vi "Sub01_CommandBuilder - Copy.vi"(8 "error in (no error)":errorcluster, 9 "CommandInfo":T1={"RedBall"={"Min"={"G"=0, "B"=0, "R"=160}, "Max"={"G"=160, "B"=160, "R"=255}}, "YellowBall"={"Min"={"G"=140, "B"=0, "R"=140}, "Max"={"G"=255, "B"=175, "R"=255}}, "WhiteBall"={"Min"={"G"=100, "B"=100, "R"=100}, "Max"={"G"=255, "B"=255, "R"=255}}, "BallDiameter"=11, "BackGround"={"Min"={"G"=91, "B"=202, "R"=39}, "Max"={"G"=116, "B"=255, "R"=62}}, "Border"={"Min"={"G"=0, "B"=121, "R"=0}, "Max"={"G"=42, "B"=126, "R"=14}}}, 10 "filenames":string[](array[string]), 11 "path in":path) -> (0 "error out":errorcluster, 3 "String":string)   [LabVIEW 2019]
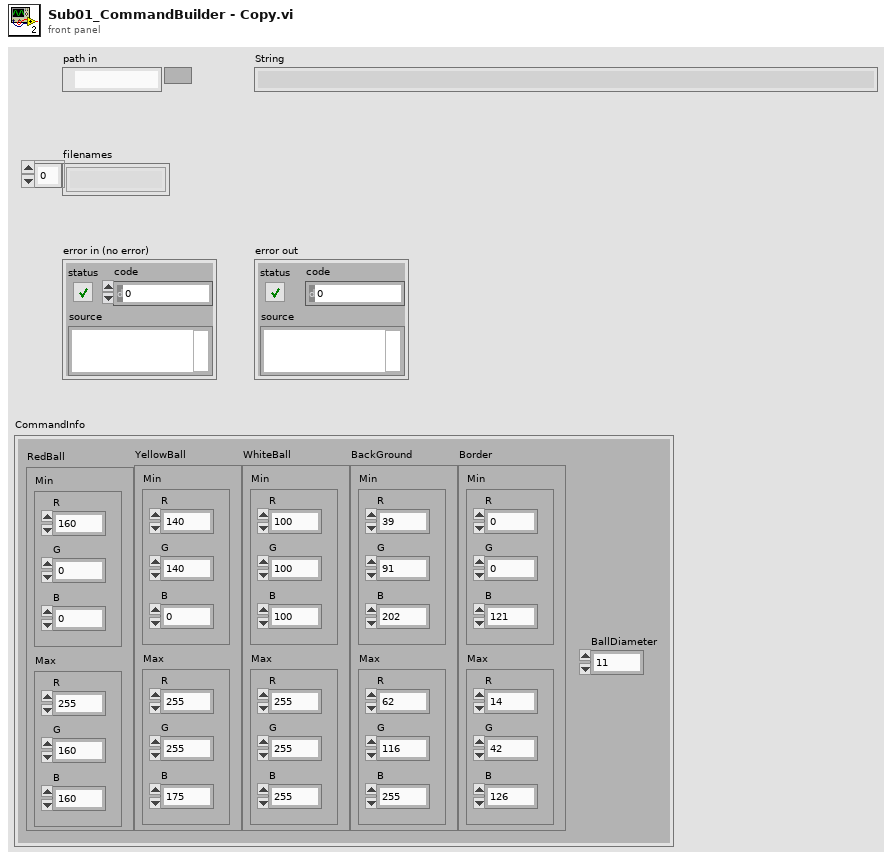
[diagram p1: front panel]
types:
  T1 = cluster{"RedBall":cluster{"Min":cluster{"G":u32, "B":u32, "R":u32}, "Max":cluster{"G":u32, "B":u32, "R":u32}}, "YellowBall":cluster{"Min":cluster{"G":u32, "B":u32, "R":u32}, "Max":cluster{"G":u32, "B":u32, "R":u32}}, "WhiteBall":cluster{"Min":cluster{"G":u32, "B":u32, "R":u32}, "Max":cluster{"G":u32, "B":u32, "R":u32}}, "BallDiameter":u32, "BackGround":cluster{"Min":cluster{"G":u32, "B":u32, "R":u32}, "Max":cluster{"G":u32, "B":u32, "R":u32}}, "Border":cluster{"Min":cluster{"G":u32, "B":u32, "R":u32}, "Max":cluster{"G":u32, "B":u32, "R":u32}}}
  T2 = cluster{"left":u32, "top":u32, "right":u32, "bottom":u32}
  T3 = typedef "imagedata.ctl" = cluster{"image type":i32, "image depth":i32, "image":u8[], "mask":u8[], "colors":u32[], "Rectangle":cluster{"left":i16, "top":i16, "right":i16, "bottom":i16}}
  T4 = cluster{"Min":cluster{"G":u32, "B":u32, "R":u32}, "Max":cluster{"G":u32, "B":u32, "R":u32}}
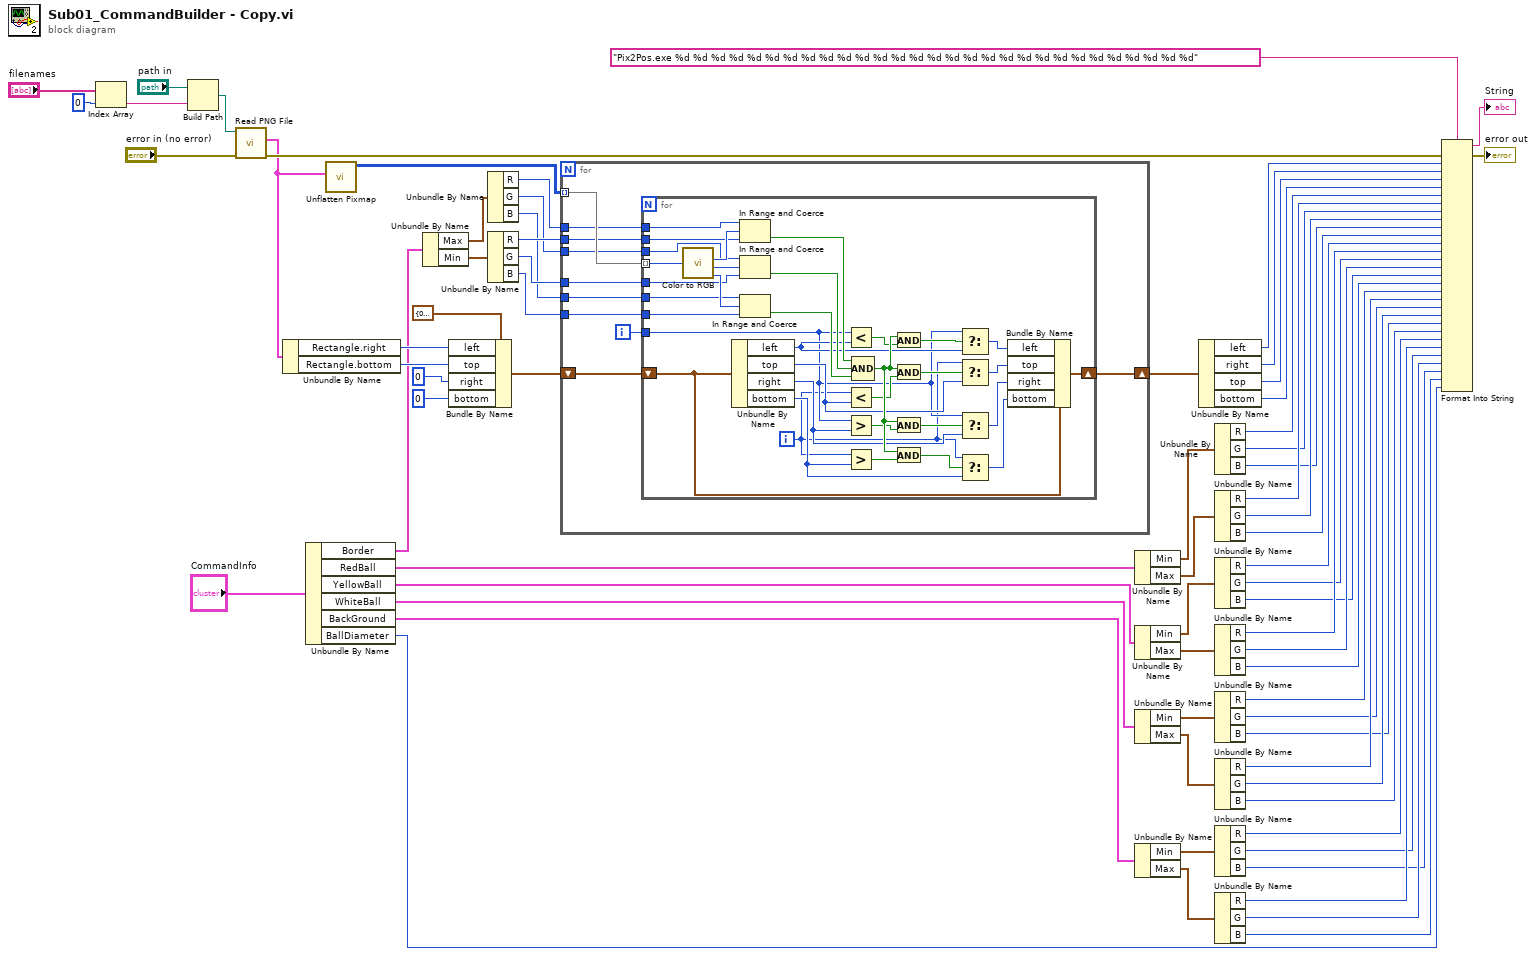
[diagram p0: block diagram]
diagram:
  n1 = Index Array(array="filenames", index=0) -> (element=w56:string)
  n2 = Build Path(base path="path in", name or relative path=w56) -> (appended path=w57:path)
  n3 = call <vilib>:"Read PNG File.vi"("error in (no error)"="error in (no error)", "path to PNG file"=w57) -> ("error out"=w59:errorcluster, "image data"=w58:T3)  [unwired: 7 in, 1 out]
  n4 = Unbundle By Name(w58) -> ("Rectangle.right"=w66:i16, "Rectangle.bottom"=w67:i16)
  n5 = Unbundle By Name("CommandInfo") -> ("Border"=w2:T4, "RedBall"=w46:T4, "YellowBall"=w39:T4, "WhiteBall"=w38:T4, "BackGround"=w29:T4, "BallDiameter"=w1:u32)
  n6 = call <vilib>:"Unflatten Pixmap.vi"("image data"=w58) -> ("24-bit pixmap"=w70:u32[][])  [unwired: 4 in, 6 out]
  n7 = Unbundle By Name(w2) -> ("Max"=w4:cluster{"G":u32, "B":u32, "R":u32}, "Min"=w3:cluster{"G":u32, "B":u32, "R":u32})
  n8 = Bundle By Name(cluster=T2 {"left"=0, "top"=0, "right"=0, "bottom"=0} ("Cluster"), "left"=w66, "top"=w67, "right"=u32 0, "bottom"=u32 0) -> (w63:T2)
  n9 = Unbundle By Name(w4) -> ("R"=w7:u32, "G"=w6:u32, "B"=w5:u32)
  n10 = Unbundle By Name(w3) -> ("R"=w10:u32, "G"=w9:u32, "B"=w8:u32)
  n11 = for {
    tunnel: w70 -> [w80] mode=indexing
    shift-right: [w77] -> w69
    shift-left: w63 -> [w79]
    tunnel: w10 -> [w76]
    tunnel: w9 -> [w75]
    tunnel: w8 -> [w74]
    tunnel: w7 -> [w73]
    tunnel: w6 -> [w72]
    tunnel: w5 -> [w71]
    i -> [w78]
    n12 = for {
      tunnel: w80 -> [w100] mode=indexing
      tunnel: w78 -> [w88]
      shift-right: [w106] -> w77
      shift-left: w79 -> [w107]
      tunnel: w76 -> [w86]
      tunnel: w75 -> [w85]
      tunnel: w74 -> [w84]
      tunnel: w73 -> [w83]
      tunnel: w72 -> [w82]
      tunnel: w71 -> [w81]
      i -> [w87]
      n13 = call <vilib>:"Color to RGB.vi"("Color"=w100) -> ("R"=w95:u8, "G"=w94:u8, "B"=w93:u8)  [unwired: 1 out]
      n14 = Unbundle By Name(w107) -> ("left"=w92:u32, "top"=w91:u32, "right"=w90:u32, "bottom"=w89:u32)
      n15 = In Range and Coerce(upper limit=w83, x=w95, lower limit=w86) -> (In Range?=w98:bool)  [unwired: 1 out]
      n16 = In Range and Coerce(upper limit=w82, x=w94, lower limit=w85) -> (In Range?=w97:bool)  [unwired: 1 out]
      n17 = In Range and Coerce(upper limit=w81, x=w93, lower limit=w84) -> (In Range?=w96:bool)  [unwired: 1 out]
      n18 = Less?(x=w88, y=w92) -> (x < y?=w104:bool)
      n19 = Less?(x=w87, y=w91) -> (x < y?=w103:bool)
      n20 = Greater?(x=w88, y=w90) -> (0:w102:bool)
      n21 = Greater?(x=w87, y=w89) -> (0:w101:bool)
      n22 = Compound Arithmetic op=AND(w98, w97, w96) -> (w105:bool)
      n23 = And(x=w105, y=w104) -> (x .and. y?=w110:bool)
      n24 = And(x=w105, y=w103) -> (x .and. y?=w109:bool)
      n25 = And(x=w105, y=w102) -> (x .and. y?=w99:bool)
      n26 = And(x=w105, y=w101) -> (x .and. y?=w108:bool)
      n27 = Select(t=w88, s=w110, f=w92) -> (s? t:f=w114:u32)
      n28 = Select(t=w87, s=w109, f=w91) -> (s? t:f=w113:u32)
      n29 = Select(t=w88, s=w99, f=w90) -> (s? t:f=w112:u32)
      n30 = Select(t=w87, s=w108, f=w89) -> (s? t:f=w111:u32)
      n31 = Bundle By Name(cluster=w107, "left"=w114, "top"=w113, "right"=w112, "bottom"=w111) -> (w106:T2)
    }
  }
  n32 = Unbundle By Name(w46) -> ("Min"=w45:cluster{"G":u32, "B":u32, "R":u32}, "Max"=w44:cluster{"G":u32, "B":u32, "R":u32})
  n33 = Unbundle By Name(w39) -> ("Min"=w43:cluster{"G":u32, "B":u32, "R":u32}, "Max"=w42:cluster{"G":u32, "B":u32, "R":u32})
  n34 = Unbundle By Name(w38) -> ("Min"=w41:cluster{"G":u32, "B":u32, "R":u32}, "Max"=w40:cluster{"G":u32, "B":u32, "R":u32})
  n35 = Unbundle By Name(w29) -> ("Min"=w31:cluster{"G":u32, "B":u32, "R":u32}, "Max"=w30:cluster{"G":u32, "B":u32, "R":u32})
  n36 = Unbundle By Name(w69) -> ("left"=w51:u32, "right"=w50:u32, "top"=w49:u32, "bottom"=w48:u32)
  n37 = Unbundle By Name(w45) -> ("R"=w37:u32, "G"=w35:u32, "B"=w33:u32)
  n38 = Unbundle By Name(w44) -> ("R"=w36:u32, "G"=w34:u32, "B"=w32:u32)
  n39 = Unbundle By Name(w43) -> ("R"=w28:u32, "G"=w26:u32, "B"=w24:u32)
  n40 = Unbundle By Name(w42) -> ("R"=w27:u32, "G"=w25:u32, "B"=w23:u32)
  n41 = Unbundle By Name(w41) -> ("R"=w22:u32, "G"=w20:u32, "B"=w18:u32)
  n42 = Unbundle By Name(w40) -> ("R"=w21:u32, "G"=w19:u32, "B"=w17:u32)
  n43 = Unbundle By Name(w31) -> ("R"=w16:u32, "G"=w14:u32, "B"=w12:u32)
  n44 = Unbundle By Name(w30) -> ("R"=w15:u32, "G"=w13:u32, "B"=w11:u32)
  n45 = Format Into String(format string="Pix2Pos.exe %d %d %d %d %d %d %d %d %d %d %d %d %d %d %d %d %d %d %d %d %d %d %d %d %d %d %d %d %d", error in=w59, w51, w50, w49, w48, w37, w36, w35, w34, w33, w32, w28, w27, w26, w25, w24, w23, w22, w21, w20, w19, w18, w17, w16, w15, w14, w13, w12, w11, w1) -> (resulting string=→"String":string, error out=→"error out":errorcluster)  [unwired: 1 in]
